vi "HTTP_Save.vi"(8 "error in (no error)":errorcluster, 10 "Code":string, 11 "Name":string="file.py") -> (0 "error out":errorcluster, 3 "PUT Code":T1)   [LabVIEW 2020]
uses:
  RestAPI.ctl
  JSON_Formats.vi
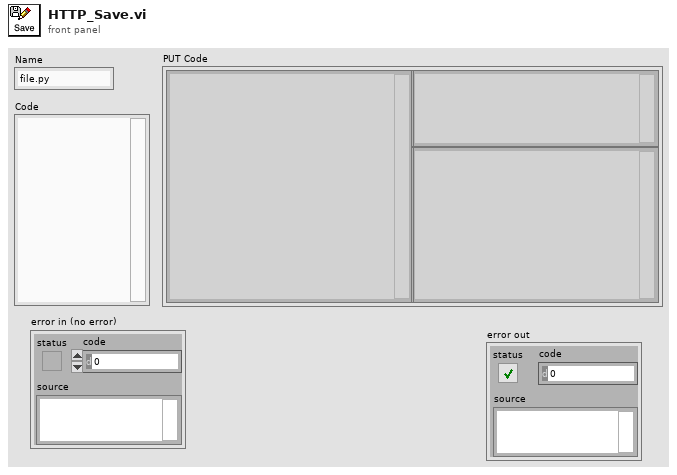
[diagram p1: front panel]
types:
  T1 = typedef "RestAPI.ctl" = cluster{"headers 2":string, "headers":string, "body":string}
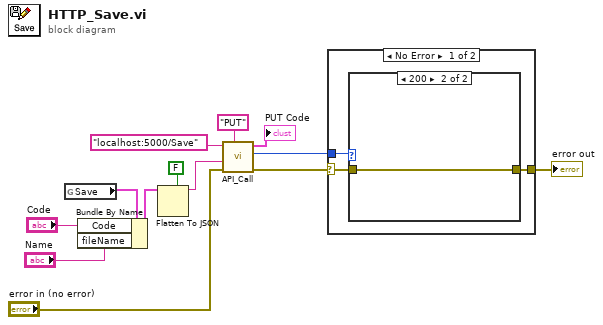
[diagram p0: block diagram]
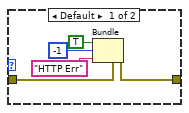
[diagram p2: hidden frame]
diagram:
  n1 = global read "JSON_Formats.vi" "Save"() -> (w3:cluster{"fileName":string, "Code":string})
  n2 = Bundle By Name(cluster=w3, "Code"="Code", "fileName"="Name") -> (w10:cluster{"fileName":string, "Code":string})
  n3 = Flatten To JSON(enable LabVIEW extensions? (T)=FALSE, anything=w10) -> (JSON string=w5:string)  [unwired: 1 in, 1 out]
  n4 = call "API_Call.vi"("Cmd"="PUT" ("input 1"), "error in (no error)"="error in (no error)", "JSON string"=w5, "url"="localhost:5000/Save") -> ("error out"=w11:errorcluster, "Err Code"=w12:i32, "Communication"=→"PUT Code":T1)  [unwired: 5 in]
  n5 = case shown="No Error" w11 {
    selector: w11 -> [w15 w23]
    tunnel: w12 -> [w16 _]
    tunnel: [w14 w23] -> w13
    frame No Error {
      n6 = case shown="200" w16 {
        tunnel: w15 -> [w21 w22]
        tunnel: [w20 w22] -> w14
        frame Default {
          n7 = Bundle(cluster=w21, "status"=TRUE, "code"=-1, "source"="HTTP Err") -> (w20:errorcluster)
        }
        frame 200 {
        }
      }
    }
    frame Error {
    }
  }
  "error out" <- w13
